vi "ReadQ.vi"(8 "error in (no error)":errorcluster, 11 "timeout in ms (200)":i32=200) -> (0 "error out":errorcluster, 2 "Variant":variant, 3 "State":T1=enum."Error")   [LabVIEW 2017, in "WebRead.lvlib"]
doc: "Read data from main coms Q"
uses:
  WebRead.lvlib
  ctl/MainStates.ctl
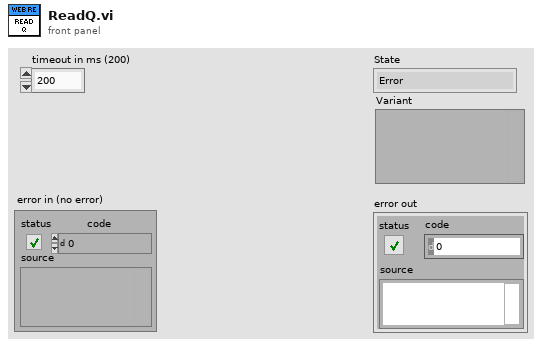
[diagram p1: front panel]
types:
  T1 = typedef "WebRead.lvlib/MainStates.ctl" = enum16{"Timeout", "Error", "Exit", "Init"}
  T2 = typedef "Temp.lvlib/MainData.ctl" = cluster{"State":T3, "Variant":variant}
  T3 = typedef "Temp.lvlib/MainStates.ctl" = enum16{"Timeout", "Error", "Exit", "Init"}
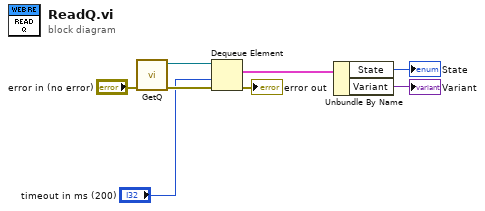
[diagram p0: block diagram]
diagram:
  n1 = call "GetQ.vi"("error in (no error)"="error in (no error)") -> ("error out"=w7:errorcluster, "Q out"=w8:refnum<queue>)  [unwired: 9 in]
  n2 = Dequeue Element(queue=w8, timeout in ms (-1)="timeout in ms (200)", error in (no error)=w7) -> (element=w4:T2, error out=→"error out":errorcluster)  [unwired: 2 out]
  n3 = Unbundle By Name(w4) -> ("State"=→"State":T3, "Variant"=→"Variant":variant)
